vi "SPI-MAX6675 Thermocouple.vi"() -> ()   [LabVIEW 2014]
doc: "This example shows how to read the temperature from a MAX6675 SPI K-Type Thermocouple to Digital converter. The temperature is read in Celsius, then converted to Fahrenheit and written to the serial port every 200ms. On AVR targets only one Chip Select pin (pin 10) is supported by the SPI peripheral, however on Due targets, other CS Pins can be selected on the front panel before downloading."
uses:
  <vilib>/Aledyne-TSXperts/Arduino Compatible Compiler for LabVIEW/Code Generator/Arduino APIs/SPI/SPI Bit Order.ctl
  <vilib>/Aledyne-TSXperts/Arduino Compatible Compiler for LabVIEW/Code Generator/Arduino APIs/SPI/SPI Data Mode.ctl
  <vilib>/Aledyne-TSXperts/Arduino Compatible Compiler for LabVIEW/Code Generator/Arduino APIs/Serial/Serial Settings.ctl
  <vilib>/Aledyne-TSXperts/Arduino Compatible Compiler for LabVIEW/Code Generator/Arduino APIs/SPI/SPI Transfer Mode.ctl
  <vilib>/Aledyne-TSXperts/Arduino Compatible Compiler for LabVIEW/Arduino Compatible Compiler for LabVIEW.lvlib
panel:
  out "Data Read":u8
  # "Overview: Demonstrates how to acquire temperature data from a MAX6675 SPI K-Type thermocouple to digital converter connected to the SPI peripheral of an Arduino target.\n\nInstructions:\n1. Wire a MAX6675 to the SPI peripheral pins of the Arduino target as shown below.\n2. Wire a K-Type thermocouple to the MAX6675 board.\n3.  Open Tools>Arduino Compatible Compiler for LabVIEW in LabVIEW, then select File>Load VI, and select this VI and then Compile and Download.\n4. Once downloaded, open a serial connection to the Arduino board and observe the temperature data being acquired."
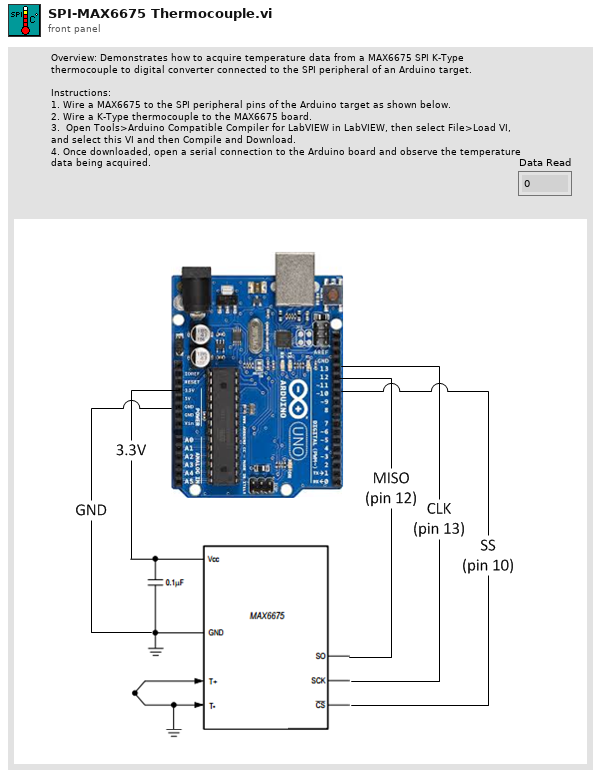
[diagram p1: front panel]
types:
  T1 = typedef "Arduino Compatible Compiler for LabVIEW.lvlib/Serial Settings.ctl" = u16
  T2 = typedef "Arduino Compatible Compiler for LabVIEW.lvlib/SPI Data Mode.ctl" = enum16{"Mode 0", "Mode 1", "Mode 2", "Mode 3"}
  T3 = typedef "Arduino Compatible Compiler for LabVIEW.lvlib/SPI Bit Order.ctl" = enum16{"LSB First", "MSB First"}
  T4 = typedef "Arduino Compatible Compiler for LabVIEW.lvlib/SPI Transfer Mode.ctl" = enum16{"Continue", "Last"}
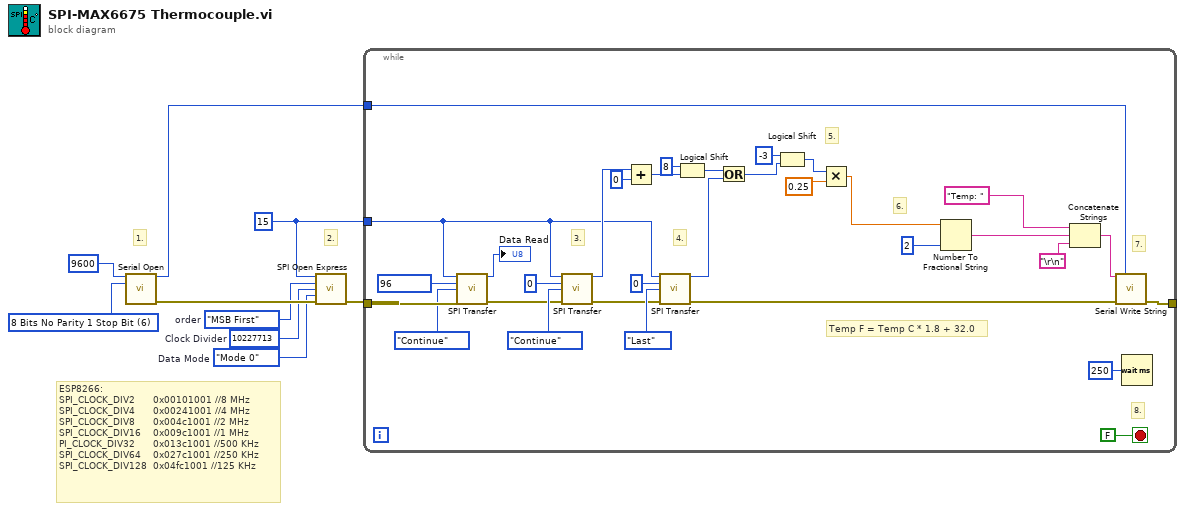
[diagram p0: block diagram]
diagram:
  w4 = u8 15 ("CS Pin")
  w2 = u32 10227713  # Clock Divider
  w7 = T1 6 items=["5 Bits No Parity 1 Stop Bit"=0, "6 Bits No Parity 1 Stop Bit"=2, "7 Bits No Parity 1 Stop Bit"=4, "8 Bits No Parity 1 Stop Bit"=6, "5 Bits No Parity 2 Stop Bits"=8, "6 Bits No Parity 2 Stop Bits"=10, "7 Bits No Parity 2 Stop Bits"=12, "8 Bits No Parity 2 Stop Bits"=14, "5 Bits Even Parity 1 Stop Bits"=32, "6 Bits Even Parity 1 Stop Bits"=34, "7 Bits Even Parity 1 Stop Bits"=36, "8 Bits Even Parity 1 Stop Bits"=38, "5 Bits Even Parity 2 Stop Bits"=40, "6 Bits Even Parity 2 Stop Bits"=42, "7 Bits Even Parity 2 Stop Bits"=44, "8 Bits Even Parity 2 Stop Bits"=46, "5 Bits Odd Parity 1 Stop Bits"=48, "6 Bits Odd Parity 1 Stop Bits"=50, "7 Bits Odd Parity 1 Stop Bits"=52, "8 Bits Odd Parity 1 Stop Bits"=54, "5 Bits Odd Parity 2 Stop Bits"=56, "6 Bits Odd Parity 2 Stop Bits"=58, "7 Bits Odd Parity 2 Stop Bits"=60, "8 Bits Odd Parity 2 Stop Bits"=62] ("Serial Settings")
  w1 = SPI_Data_Mode."Mode 0"  # Data Mode
  w3 = SPI_Bit_Order."MSB First"  # order
  # "ESP8266:\nSPI_CLOCK_DIV2 \t   \t0x00101001 //8 MHz\nSPI_CLOCK_DIV4 \t\t   0x00241001 //4 MHz\nSPI_CLOCK_DIV8 \t\t   0x004c1001 //2 MHz\nSPI_CLOCK_DIV16 \t  0x009c1001 //1 MHz\nPI_CLOCK_DIV32    \t 0x013c1001 //500 KHz\nSPI_CLOCK_DIV64   \t0x027c1001 //250 KHz\nSPI_CLOCK_DIV128 \t0x04fc1001 //125 KHz"
  # "2."
  # "1."
  n1 = call <vilib>:"Serial Open.vi"("Speed"=u32 9600, "Serial Settings"=w7) -> ("Instance"=w8:u8, "error out"=w6:errorcluster)  [unwired: 12 in]
  n2 = call <vilib>:"SPI Open Express.vi"("CS Pin"=w4, "order"=w3, "Clock Divider"=w2, "Data Mode"=w1, "error in (no error)"=w6) -> ("error out"=w5:errorcluster)  [unwired: 10 in]
  n3 = while {
    tunnel: [w27] -> _
    tunnel: w8 -> [w34]
    tunnel: w4 -> [w13]
    tunnel: w5 -> [w15]
    stop <- FALSE stop-if-true
    # "8."
    # "7."
    # "6."
    # "5."
    # "4."
    # "3."
    # "Temp F = Temp C * 1.8 + 32.0"
    n4 = call <vilib>:"SPI Transfer.vi"("CS Pin"=w13, "Data"=u8 96, "Transfer Mode"=SPI_Transfer_Mode."Continue", "error in (no error)"=w15) -> ("Data Read"=→"Data Read":u8, "error out"=w14:errorcluster)  [unwired: 10 in]
    n5 = call <vilib>:"SPI Transfer.vi"("CS Pin"=w13, "Data"=u8 0, "Transfer Mode"=SPI_Transfer_Mode."Continue", "error in (no error)"=w14) -> ("Data Read"=w21:u8, "error out"=w39:errorcluster)  [unwired: 10 in]
    n6 = Add(x=w21, y=u16 0) -> (x+y=w37:u16)
    n7 = call <vilib>:"SPI Transfer.vi"("CS Pin"=w13, "Data"=u8 0, "Transfer Mode"=SPI_Transfer_Mode."Last", "error in (no error)"=w39) -> ("Data Read"=w20:u8, "error out"=w28:errorcluster)  [unwired: 10 in]
    n8 = Logical Shift(y=i16 8, x=w37) -> (x << y=w35:u16)
    n9 = Or(x=w35, y=w20) -> (x .or. y?=w24:u16)
    n10 = Logical Shift(y=i16 -3, x=w24) -> (x << y=w23:u16)
    n11 = Multiply(x=w23, y=0.25 ("number")) -> (x*y=w18:dbl)
    n12 = Number To Fractional String(number=w18, precision (6)=i16 2) -> (F-format string=w33:string)  [unwired: 2 in]
    n13 = Concatenate Strings("Temp: " ("string"), w33, "\r\n" ("End of Line Constant")) -> (w31:string)
    n14 = call <vilib>:"Serial Write String.vi"("String"=w31, "Instance"=w34, "error in (no error)"=w28) -> ("error out"=w27:errorcluster)  [unwired: 12 in]
    n15 = Wait (ms)(milliseconds to wait=u32 250) -> ()  [unwired: 1 out]
  }
